vi "Driftmessdaten anzeigen.vi"(9 "Spaninlet":i32, 11 "error in (no error)":errorcluster caption="Fehler (Eingang, kein Fehler)") -> (4 "Anzeigecluster":T1 {"Wert 5" format="%.3g"; "Wert 4" format="%.3g"; "Wert 3" format="%.3g"; "Wert 2" format="%.3g"; "Wert 1" format="%.3g"}, 15 "error out":errorcluster caption="Fehler (Ausgang)")   [LabVIEW 2020, in "EPA 1065.lvlib" / "Gas Analyzer Drift 1065-550.lvlib"]
uses:
  Gas Analyzer Drift 1065-550.lvlib
  Anzeigecluster.ctl
  Messdaten/Aktionen FGV Messdaten.ctl
  Seiten/FT-IR/Aktionen EVID-Codes.ctl
  Seiten/FT-IR/FGV FT-IR Aktionen.ctl
  Chiller NO2 1065-376/Aktion FGV Drift Daten.ctl
  Seiten/FT-IR/FGV FT-IR Gasliste Aktionen.ctl
  Messdaten/Gewichtung (Stichprobe).ctl
  Seiten/Gaszuordnung AO/FGV Gaszuordnung Grenzen&Einheit Aktion.ctl
  Messdaten/Messdaten.lvlib
  Seiten/FT-IR/FT-IR.lvlib
  Seiten/Gaszuordnung AO/Gaszuordnung AO.lvlib
panel:
  # "Komponente"
  # "Aktueller Wert"
  # "Einheit"
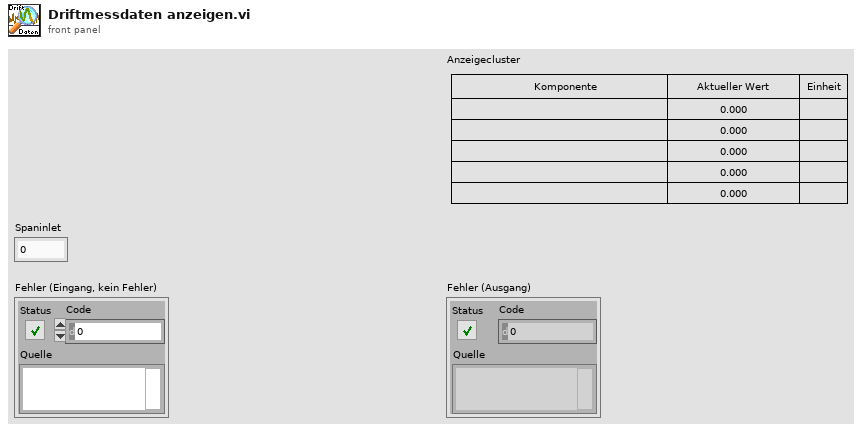
[diagram p1: front panel]
types:
  T1 = typedef "EPA 1065.lvlib/Gas Analyzer Drift 1065-550.lvlib/Anzeigecluster.ctl" = cluster{"Komponente 1":string, "Komponente 2":string, "Komponente 3":string, "Komponente 4":string, "Komponente 5":string, "Wert 1":sgl, "Wert 2":sgl, "Wert 3":sgl, "Wert 4":sgl, "Wert 5":sgl, "Einheit 1":string, "Einheit 2":string, "Einheit 3":string, "Einheit 4":string, "Einheit 5":string}
  T2 = typedef "FT-IR.lvlib/FGV FT-IR Gasliste Aktionen.ctl" = enum16{"lesen", "Gasliste FT-IR", "Gasliste ausgelesen", "laden", "speichern", "löschen"}
  T3 = typedef "EPA 1065.lvlib/Gas Analyzer Drift 1065-550.lvlib/Aktion FGV Drift Daten.ctl" = enum16{"lesen", "Konfig Daten", "PDF einstellen", "laden", "speichern", "Tabelle init", "Zeile Prüfen", "Info schreiben", "Span Einstellung", "Pre Werte schreiben", "Post Werte schreiben", "NB Pre Wert schreiben", "NB Post Wert schreiben", "Tabelle löschen"}
  T4 = typedef "FT-IR.lvlib/FGV FT-IR Aktionen.ctl" = enum16{"lesen", "NOG setzen", "NOS setzen", "Initialisieren", "speichern", "ALLES setzen", "FT-IR Spektrum loggen", "Komm Stoppen", "Spektrum LogKonfig"}
  T5 = typedef "FT-IR.lvlib/Aktionen EVID-Codes.ctl" = enum16{"lesen", "setzen", "laden", "speichern", "1Hz/5Hz", "Smoothing", "Rolling Average"}
  T6 = typedef "Messdaten.lvlib/Aktionen FGV Messdaten.ctl" = enum16{"lesen", "schreiben", "löschen", "Mittelwerte", "Komponente"}
  T7 = typedef "EPA 1065.lvlib/Gas Analyzer Drift 1065-550.lvlib/Spaninlet Cluster.ctl" = cluster{"Span Inlet Active":T8, "Analysator":T9, "Konfig Gasflasche":T8, "Gasflasche":T10, "Gasflaschen Nr.:":string, "Ablaufdatum":timestamp, "Modus":T11, "Komponenten":T12}
  T8 = typedef "System Einstellungen V2.lvlib/Konfig Gasflasche.ctl" = bool
  T9 = typedef "System Einstellungen V2.lvlib/Analysatoren.ctl" = string
  T10 = typedef "System Einstellungen V2.lvlib/Gasflasche Auswahl.ctl" = u16
  T11 = typedef "EPA 1065.lvlib/T90 Test 1065-308.lvlib/Modus.ctl" = u16
  T12 = typedef "EPA 1065.lvlib/Gas Analyzer Drift 1065-550.lvlib/Komponentencluster.ctl" = cluster{"Komponente 1":T13, "Komponente 2":T13, "Komponente 3":T13, "Komponente 4":T13, "Komponente 5":T13}
  T13 = typedef "EPA 1065.lvlib/Gas Analyzer Drift 1065-550.lvlib/Komponentenauswahl.ctl" = cluster{"Komponente:":u16, "Konzentration IST":dbl, "Einheit":enum16{"ppm", "%"}, "Genauigkeit":dbl}
  T14 = typedef "FT-IR.lvlib/1Hz-5Hz Geraet.ctl" = u16
  T15 = typedef "String - Ausgabefeld.ctl" = string
  T16 = typedef "Gaszuordnung AO.lvlib/FGV Gaszuordnung Grenzen&Einheit Aktion.ctl" = enum16{"Lesen", "Schreiben Min", "Schreiben Max", "Laden", "Speichern"}
  T17 = typedef "Messdaten.lvlib/Gewichtung (Stichprobe).ctl" = enum16{"Sample", "Population"}
  T18 = cluster{"String - Ausgabefeld":T15, "String - Ausgabefeld":T15, "String - Ausgabefeld":T15, "String - Ausgabefeld":T15, "String - Ausgabefeld":T15, "Mittelwert":sgl, "Mittelwert":sgl, "Mittelwert":sgl, "Mittelwert":sgl, "Mittelwert":sgl, "String":string, "String":string, "String":string, "String":string, "String":string}
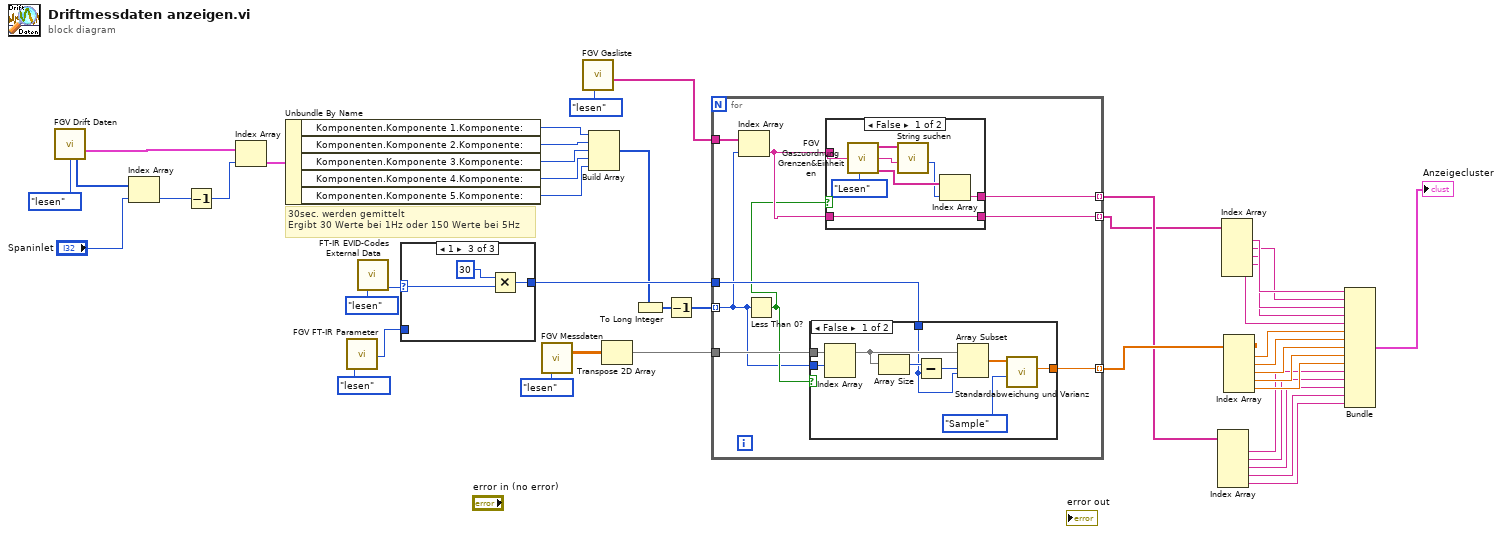
[diagram p0: block diagram]
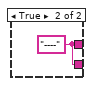
[diagram p2: hidden frame]
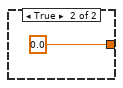
[diagram p3: hidden frame]
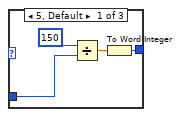
[diagram p4: hidden frame]
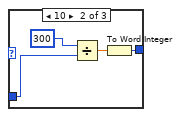
[diagram p5: hidden frame]
diagram:
  # "30sec. werden gemittelt\nErgibt 30 Werte bei 1Hz oder 150 Werte bei 5Hz"
  n1 = call "FGV Drift Daten.vi"("Aktion"=Aktion_FGV_Drift_Daten."lesen") -> ("Spangaseinstellungen"=w21:T7[], "Verwendete Spangaseingänge"=w4:i32[])  [unwired: 7 in, 6 out]
  n2 = Index Array(array=w4, index="Spaninlet") -> (element=w2:i32)
  n3 = Decrement(x=w2) -> (x-1=w1:i32)
  n4 = Index Array(array=w21, index=w1) -> (element=w30:T7)
  n5 = Unbundle By Name(w30) -> ("Komponenten.Komponente 1.Komponente:"=w36:u16, "Komponenten.Komponente 2.Komponente:"=w35:u16, "Komponenten.Komponente 3.Komponente:"=w34:u16, "Komponenten.Komponente 4.Komponente:"=w33:u16, "Komponenten.Komponente 5.Komponente:"=w32:u16)
  n6 = call "FGV FT-IR Parameter.vi"("Aktion"=FGV_FT-IR_Aktionen."lesen") -> ("NoOfScan"=w39:u32)  [unwired: 11 in, 7 out]
  n7 = call "FT-IR EVID-Codes External Data.vi"("Aktionen"=Aktionen_EVID-Codes."lesen") -> ("1Hz/5Hz Gerät"=w40:T14)  [unwired: 9 in, 5 out]
  n8 = case shown="1" w40 {
    selector: w40 -> [_ _ w53]
    tunnel: [w45 w49 w54] -> w37
    tunnel: w39 -> [w47 w51 _]
    frame 5, Default {
      n9 = Divide(x=150, y=w47) -> (x/y=w46:dbl)
      n10 = To Word Integer(number=w46) -> (16bit integer=w45:i16)
    }
    frame 10 {
      n11 = Divide(x=300, y=w51) -> (x/y=w50:dbl)
      n12 = To Word Integer(number=w50) -> (16bit integer=w49:i16)
    }
    frame 1 {
      n13 = Multiply(x=30, y=w53) -> (x*y=w54:i32)
    }
  }
  n14 = call "FGV Messdaten.vi"("Aktionen"=Aktionen_FGV_Messdaten."lesen") -> ("Messdaten"=w43:sgl[][])  [unwired: 6 in, 8 out]
  n15 = call "FGV Gasliste.vi"("Aktionen"=FGV_FT-IR_Gasliste_Aktionen."lesen") -> ("Aktuelle Gasliste gesamt"=w18:T15[])  [unwired: 8 in, 2 out]
  n16 = Build Array(w36, w35, w34, w33, w32) -> (w29:u16[])
  n17 = Transpose 2D Array(2D array=w43) -> (transposed array=w38:sgl[][])
  n18 = To Long Integer(number=w29) -> (32bit integer=w31:i32[])
  n19 = Decrement(x=w31) -> (x-1=w20:i32[])
  n20 = for {
    tunnel: w38 -> [w64]
    tunnel: w37 -> [w63]
    tunnel: [w62] -> w28 mode=indexing
    tunnel: w20 -> [w58] mode=indexing
    tunnel: w18 -> [w60]
    tunnel: [w57] -> w17 mode=indexing
    tunnel: [w56] -> w11 mode=indexing
    n21 = Index Array(array=w60, index=w58) -> (element=w61:T15)
    n22 = Less Than 0?(x=w58) -> (x < 0?=w59:bool)
    n23 = case shown="False" w59 {
      tunnel: w64 -> [w81 _]
      tunnel: w63 -> [w75 _]
      tunnel: [w74 sgl 0.0 ("Mittelwert")] -> w62
      tunnel: w58 -> [w73 _]
      frame False {
        n24 = Index Array(array=w81, index (row)=w73) -> (element=w77:sgl[])  [unwired: 1 in]
        n25 = Array Size(array=w77) -> (size(s)=w80:i32)
        n26 = Subtract(x=w80, y=w75) -> (x-y=w76:i32)
        n27 = Array Subset(array=w77, index=w76, length=w75) -> (w78:sgl[])
        n28 = call "Standardabweichung und Varianz.vi"("Gewichtung (Stichprobe)"=Gewichtung_(Stichprobe)."Sample", "X"=w78) -> ("Mittelwert"=w74:sgl)  [unwired: 7 in, 2 out]
      }
      frame True {
      }
    }
    n29 = case shown="False" w59 {
      tunnel: [w67 w72] -> w57
      tunnel: w61 -> [w66 _]
      tunnel: w61 -> [w65 _]
      tunnel: [w65 w72] -> w56
      frame False {
        n30 = call "FGV Gaszuordnung Grenzen&Einheiten.vi"("Aktion"=FGV_Gaszuordnung_Grenzen&Einheit_Aktion."Lesen") -> ("Einheit neu"=w70:string[], "Namen neu"=w69:string[])  [unwired: 7 in, 2 out]
        n31 = call "String suchen.vi"("Gasname"=w66, "Such-Namen"=w69) -> ("Index"=w68:i32)  [unwired: 8 in, 1 out]
        n32 = Index Array(array=w70, index=w68) -> (element=w67:string)
      }
      frame True {
        w72 = "----" ("String")
      }
    }
  }
  n33 = Index Array(array=w17) -> (element #1=w16:string, element #2=w15:string, element #3=w14:string, element #4=w13:string, element #5=w12:string)  [unwired: 5 in]
  n34 = Index Array(array=w11) -> (element #1=w10:T15, element #2=w9:T15, element #3=w8:T15, element #4=w7:T15, element #5=w6:T15)  [unwired: 5 in]
  n35 = Index Array(array=w28) -> (element #1=w27:sgl, element #2=w26:sgl, element #3=w25:sgl, element #4=w24:sgl, element #5=w23:sgl)  [unwired: 5 in]
  n36 = Bundle("String - Ausgabefeld"=w10, "String - Ausgabefeld"=w9, "String - Ausgabefeld"=w8, "String - Ausgabefeld"=w7, "String - Ausgabefeld"=w6, "Mittelwert"=w27, "Mittelwert"=w26, "Mittelwert"=w25, "Mittelwert"=w24, "Mittelwert"=w23, "String"=w16, "String"=w15, "String"=w14, "String"=w13, "String"=w12) -> (→"Anzeigecluster":T18)  [unwired: 1 in]
